vi "Write DI_DO.vi"(4 "DO tags":string[](array[string]), 6 "DO":bool[](array[boolean]), 7 "OPC UA AI list":string[](array[string]), 8 "error in (no error)":errorcluster, 9 "DI tags":string[](array[string]), 10 "DI":T1, 11 "OPC UA server refnum in":T3) -> (0 "error out":errorcluster, 3 "OPC UA server refnum out":T3)   [LabVIEW 2019, in "OPC addons.lvlib"]
uses:
  OPC addons.lvlib
  <vilib>/OPCUA/controls/OPC UA Server Refnum.ctl
  Inputs/Ctl/DI short.ctl
  Inputs/Ctl/Parameter State.ctl
  <vilib>/OPCUA/controls/Write Status.ctl
  <vilib>/OPCUA/server/Write Variant.vi
  <vilib>/OPCUA/NI OPC UA Server.lvlib
  Inputs/Inputs.lvlib
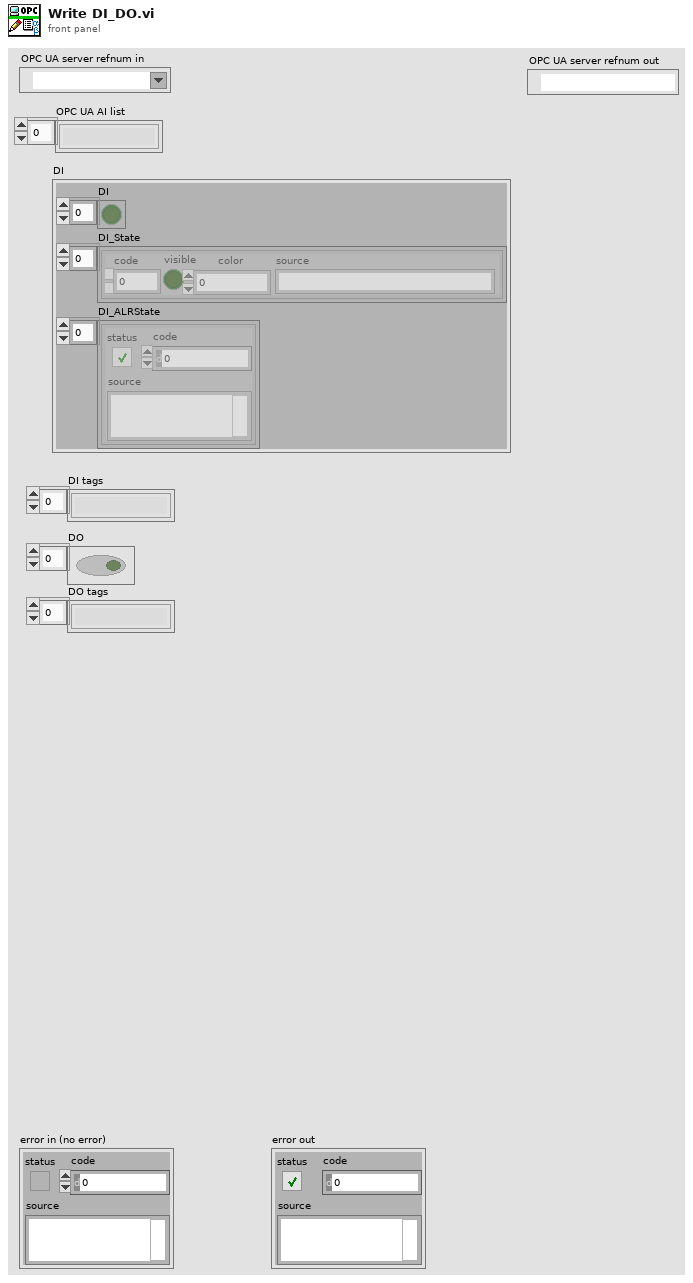
[diagram p1: front panel]
types:
  T1 = typedef "Inputs.lvlib/DI short.ctl" = cluster{"DI":bool[], "DI_State":T2[], "DI_ALRState":errorcluster[]}
  T2 = typedef "Inputs.lvlib/Parameter State.ctl" = cluster{"code":i32, "visible":bool, "color":u32, "source":string}
  T3 = typedef "OPC UA Server Refnum.ctl" = refnum<k21>
  T4 = typedef "Write Status.ctl" = u32
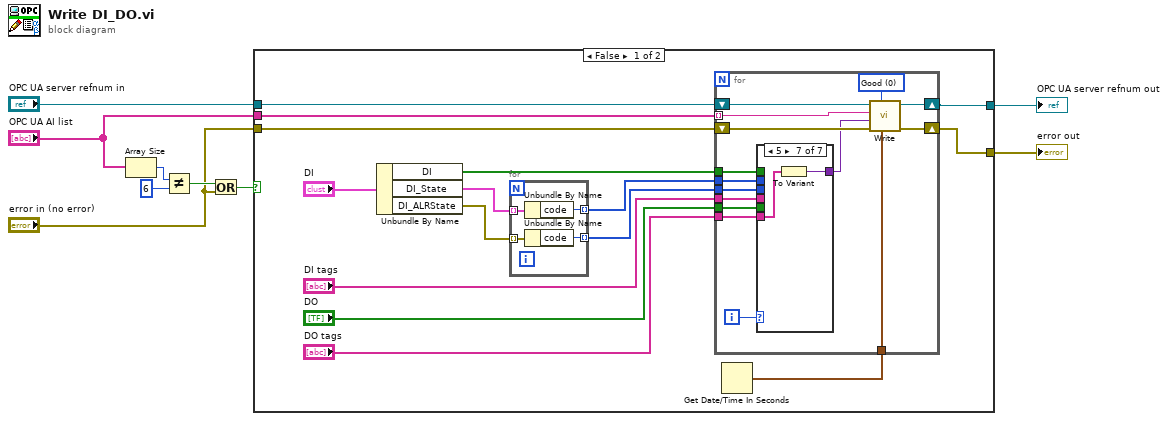
[diagram p0: block diagram]
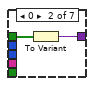
[diagram p3: hidden frame]
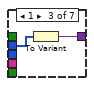
[diagram p4: hidden frame]
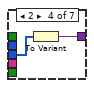
[diagram p5: hidden frame]
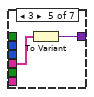
[diagram p6: hidden frame]
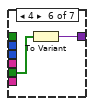
[diagram p7: hidden frame]
diagram:
  n1 = Array Size(array="OPC UA AI list") -> (size(s)=w5:i32)
  n2 = Not Equal?(x=w5, y=6) -> (x != y?=w3:bool)
  n3 = Or(x=w3, y="error in (no error)") -> (x .or. y?=w1:bool)
  n4 = case shown="False" w1 {
    tunnel: "OPC UA server refnum in" -> [w23 w57]
    tunnel: [w22 w57] -> w8
    tunnel: [w21 w56] -> w7
    tunnel: "OPC UA AI list" -> [w19 _]
    tunnel: "error in (no error)" -> [w12 w56]
    frame False {
      n5 = Unbundle By Name("DI") -> ("DI"=w14:bool[], "DI_State"=w17:T2[], "DI_ALRState"=w16:errorcluster[])
      n6 = for {
        tunnel: w17 -> [w28] mode=indexing
        tunnel: [w27] -> w15 mode=indexing
        tunnel: w16 -> [w26] mode=indexing
        tunnel: [w25] -> w11 mode=indexing
        n7 = Unbundle By Name(w28) -> ("code"=w27:i32)
        n8 = Unbundle By Name(w26) -> ("code"=w25:i32)
      }
      n9 = Get Date/Time In Seconds() -> (seconds since 1Jan1904=w24:timestamp)
      n10 = for {
        tunnel: w24 -> [w33]
        tunnel: w14 -> [w43]
        tunnel: w15 -> [w41]
        tunnel: w19 -> [w31] mode=indexing
        tunnel: w11 -> [w40]
        tunnel: "DI tags" -> [w39]
        tunnel: "DO" -> [w38]
        tunnel: "DO tags" -> [w37]
        shift-right: [w30] -> w22
        shift-left: w23 -> [w35]
        shift-right: [w29] -> w21
        shift-left: w12 -> [w34]
        i -> [w42]
        w36 = T4 0 items=["Good"=0, "Uncertain"=1073741824, "Uncertain_InitialValue"=1083310080, "Uncertain_LastUsableValue"=1083179008, "Uncertain_SensorNotAccurate"=1083375616, "Uncertain_EngineeringUnitsExceeded"=1083441152, "Bad"=2147483648, "Bad_NoCommunication"=2150694912, "Bad_NotReadable"=2151284736, "Bad_NotWritable"=2151350272, "Bad_OutOfRange"=2151415808, "Bad_WaitingForInitialData"=2150760448] ("node status")
        n11 = case shown="5" w42 {
          tunnel: w43 -> [_ w45 _ _ _ _ _]
          tunnel: [_ w44 w47 w49 w51 w53 w55] -> w32
          tunnel: w41 -> [_ _ w46 _ _ _ _]
          tunnel: w40 -> [_ _ _ w48 _ _ _]
          tunnel: w39 -> [_ _ _ _ w50 _ _]
          tunnel: w38 -> [_ _ _ _ _ w52 _]
          tunnel: w37 -> [_ _ _ _ _ _ w54]
          frame -1, Default {
          }
          frame 0 {
            n12 = To Variant(anything=w45) -> (Variant=w44:variant)
          }
          frame 1 {
            n13 = To Variant(anything=w46) -> (Variant=w47:variant)
          }
          frame 2 {
            n14 = To Variant(anything=w48) -> (Variant=w49:variant)
          }
          frame 3 {
            n15 = To Variant(anything=w50) -> (Variant=w51:variant)
          }
          frame 4 {
            n16 = To Variant(anything=w52) -> (Variant=w53:variant)
          }
          frame 5 {
            n17 = To Variant(anything=w54) -> (Variant=w55:variant)
          }
        }
        n18 = call-poly <vilib>:"Write.vi"("timestamp (current time)"=w33, "node status"=w36, "error in (no error)"=w34, "value"=w32, "node ID"=w31, "OPC UA server refnum in"=w35) -> ("error out"=w29:errorcluster, "OPC UA server refnum out"=w30:T3)  [unwired: 3 in, 1 out]
      }
    }
    frame True {
    }
  }
  "OPC UA server refnum out" <- w8
  "error out" <- w7
